vi "Get Roller Orientation.vi"(8 "error in (no error)":errorcluster, 11 "mecanum wheel in":refnum<class "NI_Robotics_Mecanum Wheel.lvclass">) -> (0 "error out":errorcluster, 2 "roller orientation":T1 items=["Left", "Right"], 3 "mecanum wheel out":refnum<class "NI_Robotics_Mecanum Wheel.lvclass">)   [LabVIEW 2017, in "NI_Robotics_Mecanum Wheel.lvclass"]
uses:
  <vilib>/robotics/Steering/Mecanum Wheel/NI_Robotics_Mecanum Wheel.lvclass
  <vilib>/robotics/Steering/Mecanum Wheel/Roller Orientation.ctl
  <vilib>/robotics/Steering/Mecanum Wheel/NI_Robotics_Mecanum Wheel.lvclass/NI_Robotics_Mecanum Wheel.ctl
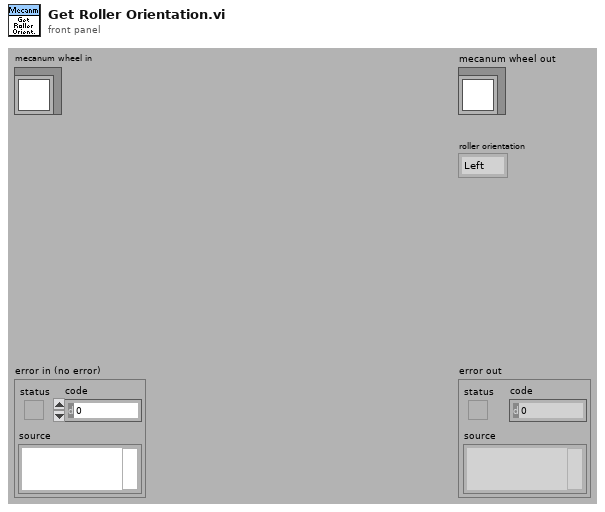
[diagram p1: front panel]
types:
  T1 = typedef "NI_Robotics_Mecanum Wheel.lvclass/Roller Orientation.ctl" = u16
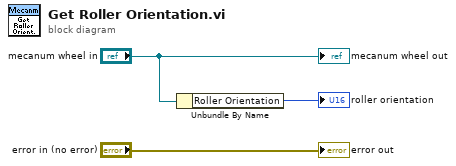
[diagram p0: block diagram]
diagram:
  n1 = Unbundle By Name("mecanum wheel in") -> ("Roller Orientation"=→"roller orientation":T1)
  "error out" <- "error in (no error)"
  "mecanum wheel out" <- "mecanum wheel in"
